vi "final project vi (imman).vi"() -> ()   [LabVIEW 2020]
panel:
  out "Input data":dbl
  out "Output Angle":dbl
  in  "Vin 2":dbl
  in  "Vin 1":dbl
  in  "Angle 2":dbl
  in  "Angle 1 Angle 1":dbl
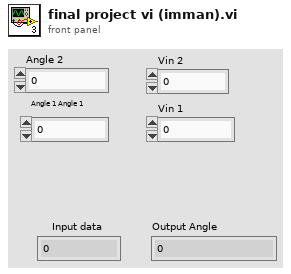
[diagram p1: front panel]
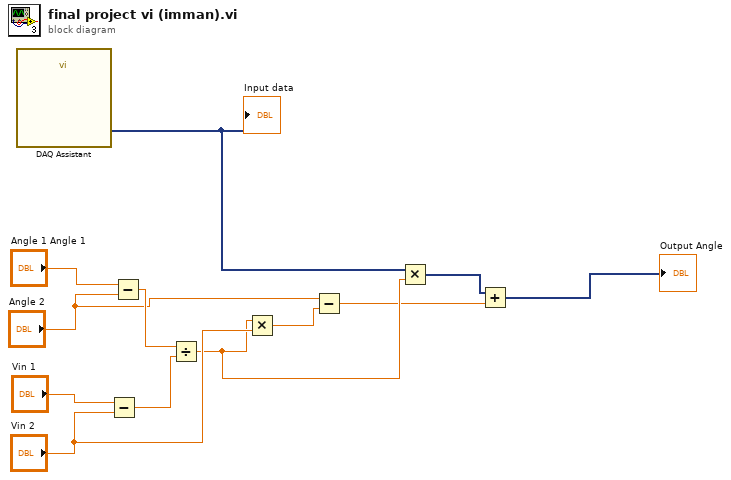
[diagram p0: block diagram]
diagram:
  n1 = call "DAQ Assistant"() -> ("data"=w1:dynamicdata)  [unwired: 16 in, 3 out]
  "Input data" <- w1
  n2 = Subtract(x="Vin 1", y="Vin 2") -> (x-y=w9:dbl)
  n3 = Subtract(x="Angle 1 Angle 1", y="Angle 2") -> (x-y=w10:dbl)
  n4 = Divide(x=w10, y=w9) -> (x/y=w5:dbl)
  n5 = Multiply(x=w5, y="Vin 2") -> (x*y=w7:dbl)
  n6 = Subtract(x="Angle 2", y=w7) -> (x-y=w3:dbl)
  n7 = Multiply(x=w1, y=w5) -> (x*y=w4:dynamicdata)
  n8 = Add(x=w4, y=w3) -> (x+y=→"Output Angle":dynamicdata)
